vi "Result_Test.vi"(8 "error in (no error)":errorcluster caption="entrée d'erreur (pas d'erreur)", 11 "Get_Voltage en entrée":refnum<class "P2056_Get_PoP.lvclass">) -> (0 "error out":errorcluster caption="sortie d'erreur", 3 "Get_Voltage en sortie":refnum<class "P2056_Get_PoP.lvclass">)   [LabVIEW 2020, in "Library Test.lvlib" / "P2056_Get_PoP.lvclass"]
uses:
  P2056_Get_PoP.lvclass
  C:/Users/ngarcin/OneDrive - Altyor/Standard TB/Suite TB45/Class/Test/Test (Default)/Test (Default).lvclass
  Commun VI/TypeDef/Variable Printable.ctl
  JSON API/JSON Value/Set from JSON string.vi
  JSON API/JSON Value/JSON Value.lvclass
  P2056_Send_Command_UART.lvclass
  JSON API/Variant JSON/Variant JSON.lvlib
  JSON API/Get Polymorphic/JSON GetSet.lvlib
  Commun VI/Library Commun.lvlib
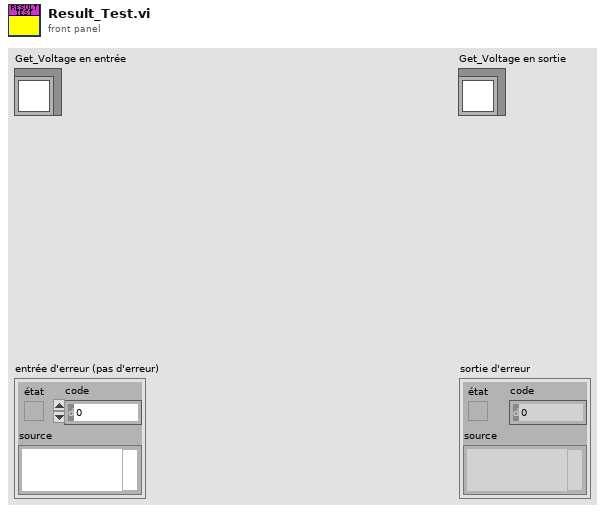
[diagram p1: front panel]
types:
  T1 = typedef "Variable Printable.ctl" = string
  T2 = enum16{"Get Variable", "Get All Variables", "Set Variable", "Delete Variable", "Delete All Variable"}
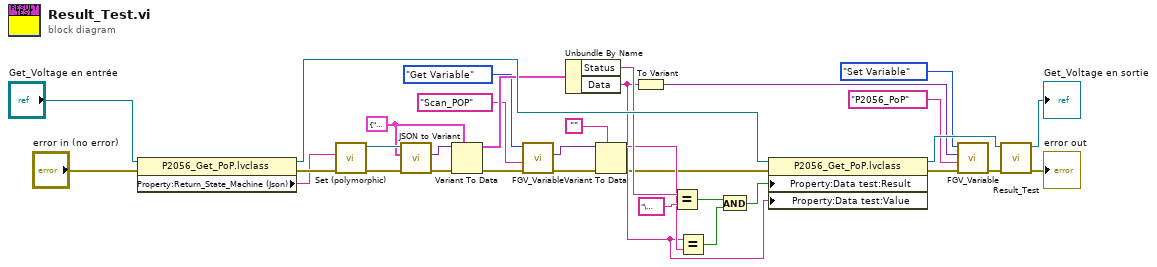
[diagram p0: block diagram]
diagram:
  w26 = cluster{"Data":string, "Status":string} {"Data"="", "Status"=""}
  n1 = property class="P2056_Get_PoP.lvclass"(reference="Get_Voltage en entrée", error in="error in (no error)") -> (reference out=w31:refnum<class "P2056_Get_PoP.lvclass">, error out=w25:errorcluster, "Property:Return_State_Machine (Json)"=w24:string)
  n2 = call-poly "Set (polymorphic).vi"("error in (no error)"=w25, "JSON stream"=w24) -> ("error out"=w28:errorcluster, "JSON Value out"=w30:refnum<class "JSON Value.lvclass">)  [unwired: 7 in, 1 out]
  n3 = call "JSON to Variant.vi"("error in (no error)"=w28, "Variant (Data Type)"=w26, "JSON Value"=w30) -> ("error out"=w29:errorcluster, "Variant out"=w27:variant)  [unwired: 7 in]
  n4 = Variant To Data(error in=w29, type=w26, Variant=w27) -> (data=w23:cluster{"Data":string, "Status":string}, error out=w2:errorcluster)
  n5 = call "FGV_Variable.vi"("error in (no error)"=w2, "Variable"=T1 "Scan_POP", "Function"=T2."Get Variable") -> ("error out"=w9:errorcluster, "Data Out"=w8:variant)  [unwired: 6 in, 1 out]
  n6 = Unbundle By Name(w23) -> ("Status"=w22:string, "Data"=w5:string)
  n7 = Variant To Data(error in=w9, type="", Variant=w8) -> (data=w6:string, error out=w1:errorcluster)
  n8 = To Variant(anything=w5) -> (Variant=w17:variant)
  n9 = Equal?(x=w22, y="\u0000") -> (x = y?=w7:bool)
  n10 = Equal?(x=w5, y=w6) -> (x = y?=w4:bool)
  n11 = And(x=w7, y=w4) -> (x .and. y?=w3:bool)
  n12 = property class="P2056_Get_PoP.lvclass"(reference=w31, error in=w1, "Property:Data test:Result"=w3, "Property:Data test:Value"=w5) -> (reference out=w18:refnum<class "P2056_Get_PoP.lvclass">, error out=w14:errorcluster)
  n13 = call "FGV_Variable.vi"("error in (no error)"=w14, "Variable"=T1 "P2056_PoP", "Data In"=w17, "Function"=T2."Set Variable") -> ("error out"=w13:errorcluster)  [unwired: 5 in, 2 out]
  n14 = call-parent "Result_Test.vi"("error in (no error)"=w13, "Get_Voltage en entrée"=w18) -> ("error out"=→"error out":errorcluster, "Get_Voltage en sortie"=→"Get_Voltage en sortie":refnum<class "P2056_Get_PoP.lvclass">)  [unwired: 8 in]
